vi "ToRepo.vi"(8 "error in":errorcluster, 9 "to repo cluster":T1, 10 "repository in":refnum<class "NISE_CEF_Repository.lvclass">, 11 "cRIO in":refnum<class "can port.lvclass">) -> (0 "error out":errorcluster, 2 "repository out":refnum<class "NISE_CEF_Repository.lvclass">, 3 "cRIO out":refnum<class "can port.lvclass">)   [LabVIEW 2013, in "can port.lvclass"]
uses:
  can port.lvclass
  <vilib>/NI/Configuration Framework/Repository/NISE_CEF_Repository.lvclass
  <vilib>/NI/Configuration Framework/Node/ToRepoCluster.ctl
  <vilib>/NI/Configuration Framework/Node/NISE_CEF_Node.lvclass
  can port.lvclass/can port.ctl
  database file/database file.lvclass
  J1939 Library/Configuration/TypeDefs/J1939 db frame.ctl
  J1939 Library/Configuration/TypeDefs/J1939 db signal.ctl
  database file/database file.lvclass/database file.ctl
  database file/Write BaudRate.vi
  database file/Write J1939 Network Address.vi
  database file/Write Name.vi
  database file/Write frames.vi
  J1939 Library/J1939.lvlib
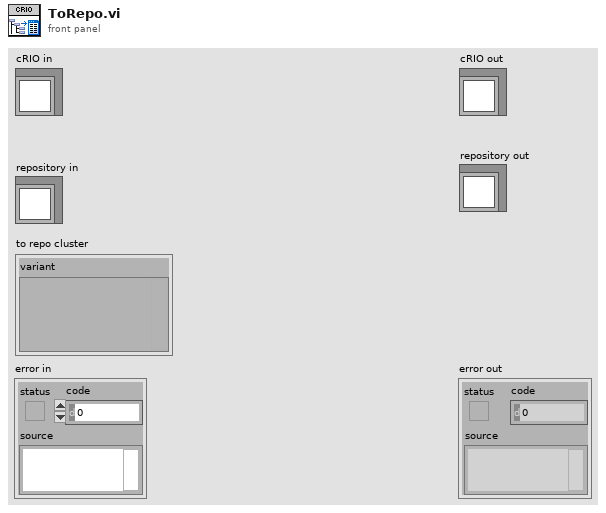
[diagram p1: front panel]
types:
  T1 = typedef "NISE_CEF_Node.lvclass/ToRepoCluster.ctl" = cluster{"variant":variant}
  T2 = typedef "J1939.lvlib/J1939 db frame.ctl" = cluster{"name":string, "Priority":u8, "PGN":u32, "Reserved Bit":u8, "Data page":u8, "PDU Format":u8, "PDU Specific":u8, "Source Address":u8, "PayldLen":u32, "signals":T3[], "Comment":string, "can timing type":u32, "transmit time":dbl, "direction":u16}
  T3 = typedef "J1939.lvlib/J1939 db signal.ctl" = cluster{"NameShort":string, "SPN":i32, "StartBit":u32, "NumBits":u32, "DataType":u32, "ByteOrdr":u32, "ScaleFac":dbl, "ScaleOff":dbl, "Max":dbl, "Min":dbl, "Default":dbl, "Unit":string, "Comment":string}
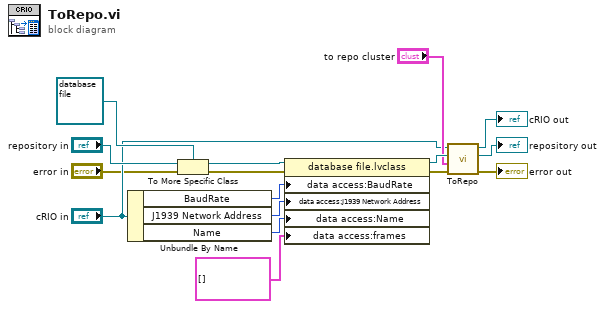
[diagram p0: block diagram]
diagram:
  n1 = Unbundle By Name("cRIO in") -> ("BaudRate"=w6:u32, "J1939 Network Address"=w2:u8, "Name"=w1:u64)
  n2 = To More Specific Class(target class=refnum<class "database file.lvclass"> refnum ("cRIO repo.lvclass"), reference="repository in", error in="error in") -> (specific class reference=w10:refnum<class "database file.lvclass">, error out=w3:errorcluster)
  n3 = property class="database file.lvclass"(reference=w10, error in=w3, "data access:BaudRate"=w6, "data access:J1939 Network Address"=w2, "data access:Name"=w1, "data access:frames"=T2[] [] ("frames")) -> (reference out=w13:refnum<class "database file.lvclass">, error out=w9:errorcluster)
  n4 = call-parent "ToRepo.vi"("error in"=w9, "to repo cluster"="to repo cluster", "repository in"=w13, "node in"="cRIO in") -> ("error out"=→"error out":errorcluster, "repository out"=→"repository out":refnum<class "NISE_CEF_Repository.lvclass">, "node out"=→"cRIO out":refnum<class "can port.lvclass">)  [unwired: 5 in]
